vi "DSF Post-Build.vi"   [LabVIEW 2017]
uses:
  Development Tools/Build Automation/Build Automation.lvlib
types:
  T1 = cluster{"Status Message":refnum<data-value>, "Progress":refnum<data-value>, "Stop":refnum<data-value>}
  T2 = enum16{"Share clones between instances", "Preallocate clone for each instance"}
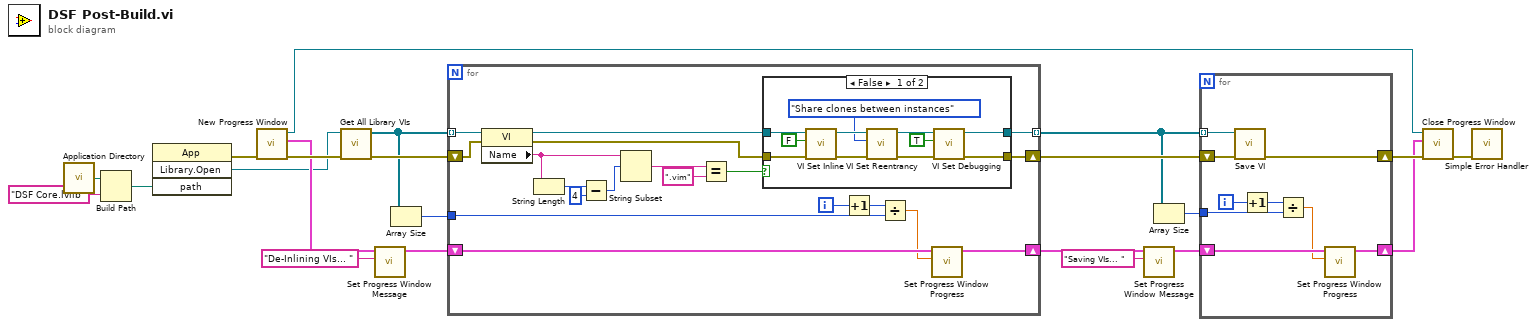
[diagram p0: block diagram]
diagram:
  n1 = call <vilib>:"Application Directory.vi"() -> ("Application Directory"=w2:path)
  n2 = Build Path(base path=w2, name or relative path="DSF Core.lvlib" ("library name")) -> (appended path=w1:path)
  n3 = invoke class="App" method="Library.Open"("path"=w1) -> (error out=w21:errorcluster, "Open Library"=w9:refnum<vi>)  [unwired: 3 in, 2 out]
  n4 = call "New Progress Window.vi"("error in (no error)"=w21) -> ("error out"=w11:errorcluster, "DVRs"=w10:T1, "VI refnum"=w15:refnum<vi>)  [unwired: 8 in]
  n5 = call "Get All Library VIs.vi"("error in (no error)"=w11, "library ref"=w9) -> ("error out"=w22:errorcluster, "vi refs"=w19:refnum<vi>[])  [unwired: 8 in]
  n6 = call "Set Progress Window Message.vi"("Status Message"="De-Inlining VIs... " ("data value"), "DVRs in"=w10) -> ("DVRs out"=w17:T1)  [unwired: 8 in, 1 out]
  n7 = Array Size(array=w19) -> (size(s)=w18:i32)
  n8 = for {
    tunnel: w19 -> [w27] mode=indexing
    shift-right: [w34] -> w14
    shift-left: w22 -> [w26]
    tunnel: w18 -> [w39]
    shift-right: [w36] -> w13
    shift-left: w17 -> [w38]
    tunnel: [w35] -> w7 mode=indexing
    i -> [w41]
    n9 = property class="VI"(reference=w27, error in=w26) -> (reference out=w25:refnum<vi>, error out=w24:errorcluster, "Name"=w33:string)
    n10 = String Length(string=w33) -> (length=w32:i32)
    n11 = Subtract(x=w32, y=4) -> (x-y=w28:i32)
    n12 = String Subset(string=w33, offset (0)=w28) -> (substring=w30:string)  [unwired: 1 in]
    n13 = Equal?(x=w30, y=".vim") -> (x = y?=w23:bool)
    n14 = case shown="False" w23 {
      tunnel: [w45 w54] -> w35
      tunnel: [w44 w53] -> w34
      tunnel: w25 -> [w43 w54]
      tunnel: w24 -> [w42 w53]
      frame False {
        n15 = call "VI Set Inline.vi"("error in (no error)"=w42, "Inline VI"=FALSE, "vi ref in"=w43) -> ("error out"=w49:errorcluster, "vi ref out"=w50:refnum<vi>)  [unwired: 7 in]
        n16 = call "VI Set Reentrancy.vi"("error in (no error)"=w49, "Reentrancy Type"=T2."Share clones between instances", "vi ref in"=w50) -> ("error out"=w46:errorcluster, "vi ref out"=w47:refnum<vi>)  [unwired: 7 in]
        n17 = call "VI Set Debugging.vi"("error in (no error)"=w46, "Allow Debugging"=TRUE, "vi ref in"=w47) -> ("error out"=w44:errorcluster, "vi ref out"=w45:refnum<vi>)  [unwired: 7 in]
      }
      frame True {
      }
    }
    n18 = Increment(x=w41) -> (x+1=w40:i32)
    n19 = Divide(x=w40, y=w39) -> (x/y=w37:dbl)
    n20 = call "Set Progress Window Progress.vi"("Progress"=w37, "DVRs in"=w38) -> ("DVRs out"=w36:T1)  [unwired: 8 in, 1 out]
  }
  n21 = call "Set Progress Window Message.vi"("Status Message"="Saving VIs... ", "DVRs in"=w13) -> ("DVRs out"=w8:T1)  [unwired: 8 in, 1 out]
  n22 = Array Size(array=w7) -> (size(s)=w6:i32)
  n23 = for {
    shift-right: [w61] -> w5
    shift-left: w14 -> [w63]
    tunnel: w7 -> [w62] mode=indexing
    shift-right: [w55] -> w4
    shift-left: w8 -> [w57]
    tunnel: w6 -> [w59]
    i -> [w58]
    n24 = call "Save VI.vi"("error in (no error)"=w63, "vi ref in"=w62) -> ("error out"=w61:errorcluster)  [unwired: 8 in, 1 out]
    n25 = Increment(x=w58) -> (x+1=w60:i32)
    n26 = Divide(x=w60, y=w59) -> (x/y=w56:dbl)
    n27 = call "Set Progress Window Progress.vi"("Progress"=w56, "DVRs in"=w57) -> ("DVRs out"=w55:T1)  [unwired: 8 in, 1 out]
  }
  n28 = call "Close Progress Window.vi"("error in (no error)"=w5, "DVRs in"=w4, "VI refnum"=w15) -> ("error out"=w16:errorcluster)  [unwired: 8 in]
  n29 = call <vilib>:"Simple Error Handler.vi"("error in (no error)"=w16) -> ()  [unwired: 4 in, 5 out]
